vi "TCP Read from Connection.vi"(5 "Options":T1={"Ignore Timeout Error"=TRUE, "timeout ms (1000)"=1000}, 7 "error in":errorcluster, 8 "index":i32) -> (0 "error out":errorcluster, 1 "Name":T2, 2 "data string":string, 4 "Timed Out?":bool)   [LabVIEW 2014, in "QwaveSys Raspberry Pi Library.lvlib"]
doc: "This VI reads an incoming package of data from the connection specified by \"index\". This VI parses the package and extracts the data name and type as described in the meta data.\n\nFor the package to be parsed correctly, the meta data must be consistent in both the sender and the receiver. The data is packaged based on the existing meta data on the sender."
uses:
  QwaveSys Raspberry Pi Library.lvlib
  _SubVIs/stm_MetaDataElement.ctl
  TCP/stm_TCP Read Options.ctl
  stm_TCPConnectionMethod.ctl
  TCP/STM Read Message (TCP).vi
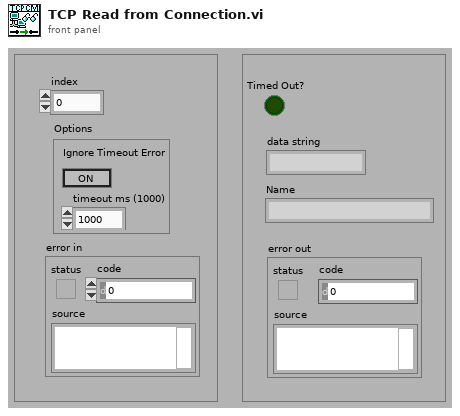
[diagram p1: front panel]
types:
  T1 = typedef "QwaveSys Raspberry Pi Library.lvlib/stm_TCP Read Options.ctl" = cluster{"Ignore Timeout Error":bool, "timeout ms (1000)":i32}
  T2 = typedef "QwaveSys Raspberry Pi Library.lvlib/stm_MetaDataElement.ctl" = string
  T3 = typedef "QwaveSys Raspberry Pi Library.lvlib/stm_TCPConnectionMethod.ctl" = enum16{"Initialize", "Add Connection", "Set Properties", "Get Connection(s)", "Remove Connection", "Remove All Connections", "Get Connection Count"}
  T4 = typedef "QwaveSys Raspberry Pi Library.lvlib/stm_TCP Connection Info.ctl" = cluster{"connection ID":refnum<k5>, "Meta data":T2[]}
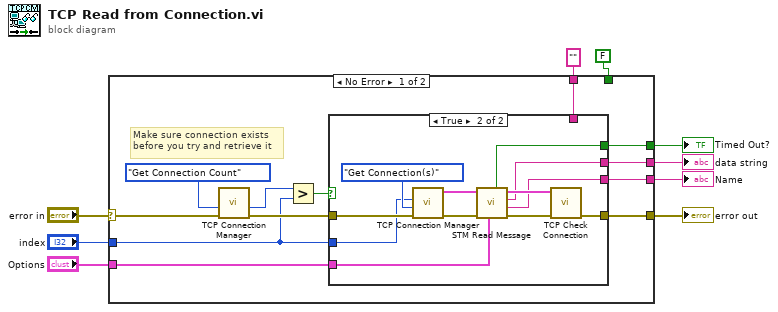
[diagram p0: block diagram]
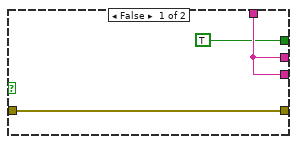
[diagram p2: hidden frame]
diagram:
  n1 = case shown="No Error" "error in" {
    selector: "error in" -> [w18 w39]
    tunnel: [w21 w39] -> w9
    tunnel: [w17 w37] -> w7
    tunnel: [w16 w38] -> w6
    tunnel: [w15 w38] -> w5
    tunnel: "" ("data string") -> [w14 w38]
    tunnel: FALSE ("Timed Out?") -> [_ w37]
    tunnel: "Options" -> [w13 _]
    tunnel: "index" -> [w11 _]
    frame No Error {
      # "Make sure connection exists\nbefore you try and retrieve it"
      n2 = call "TCP Connection Manager.vi"("error in (no error)"=w18, "Method"=stm_TCPConnectionMethod."Get Connection Count") -> ("error out"=w19:errorcluster, "Number of Connections"=w12:i32)  [unwired: 3 in, 5 out]
      n3 = Greater?(x=w12, y=w11) -> (0:w10:bool)
      n4 = case shown="True" w10 {
        tunnel: w19 -> [w24 w28]
        tunnel: [w24 w36] -> w21
        tunnel: [TRUE ("Timed Out?") w33] -> w17
        tunnel: [w23 w32] -> w16
        tunnel: [w23 w31] -> w15
        tunnel: w14 -> [w23 _]
        tunnel: w13 -> [_ w30]
        tunnel: w11 -> [_ w25]
        frame False {
        }
        frame True {
          n5 = call "TCP Connection Manager.vi"("error in (no error)"=w28, "Method"=stm_TCPConnectionMethod."Get Connection(s)", "Index"=w25) -> ("error out"=w27:errorcluster, "Connection Out"=w26:T4)  [unwired: 2 in, 5 out]
          n6 = call-poly "STM Read Message.vi"("Options"=w30, "error in"=w27, "Connection Info"=w26) -> ("error out"=w34:errorcluster, "Name"=w31:T2, "data string"=w32:string, "Connection Info Out"=w35:T4, "Timed Out?"=w33:bool)  [unwired: 2 in, 2 out]
          n7 = call "TCP Check Connection.vi"("error in (no error)"=w34, "Connection In"=w35) -> ("error out"=w36:errorcluster)  [unwired: 9 out]
        }
      }
    }
    frame Error {
    }
  }
  "error out" <- w9
  "Timed Out?" <- w7
  "data string" <- w6
  "Name" <- w5
